vi "ctx set requested device states.vi"(10 "state":u32(ring) items=["APDM_DS_RUN", "APDM_DS_HALT"], 11 "context":u32) -> (2 "function return":i32, 3 "context out":u32)   [LabVIEW 2019, in "apdm.lvlib"]
doc: "APDM_EXPORT int apdm_ctx_set_requested_device_states(apdm_ctx_t context, const enum RequestedDeviceState state);"
uses:
  apdm.lvlib
  Lee Lab/CP FES Walking 2018/Code/Working/LabVIEW/apdm.dll
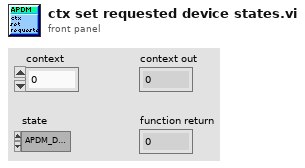
[diagram p1: front panel]
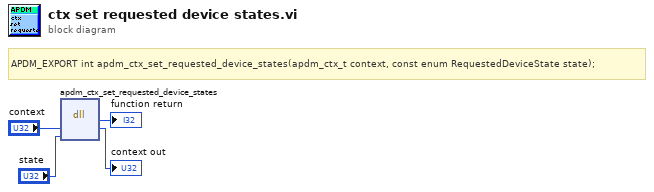
[diagram p0: block diagram]
diagram:
  # "APDM_EXPORT int apdm_ctx_set_requested_device_states(apdm_ctx_t context, const enum RequestedDeviceState state);"
  n1 = dll-call lib="C:/Users/jfalesi/Dropbox/Lee Lab/CP FES Walking 2018/Code/Working/LabVIEW/apdm.*" fn="apdm_ctx_set_requested_device_states"("context"="context", "state"="state") -> (→"function return":i32, "context"=→"context out":u32)  [unwired: 4 in, 2 out]
